vi "GUI_LiquidCrystal.vi"() -> ()   [LabVIEW 2020]
uses:
  Shared/GUI_Template/GUI_master/tcp_new_data_event.ctl
  Shared/GUI_Template/GUI_master/tcp new data cluster.ctl
panel:
  out "Film in place?":bool
  in  "User Threshold":dbl
  in  "MaxCounts::1":dbl caption="Max Counts" min=0.0 max=999999999.0
  in  "Stop":bool
  out "tcp data event":T1
  out "error IO 2":errorcluster
  in  "GUIdevice 1":string="P2-HeatCamPost"
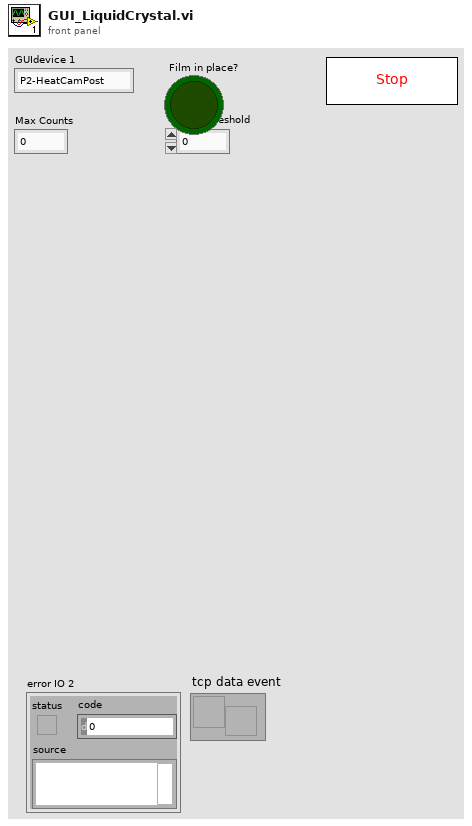
[diagram p1: front panel]
types:
  T1 = typedef "tcp_new_data_event.ctl" = refnum<user-event>
  T2 = typedef "tcp new data cluster.ctl" = cluster{"EventEnum":enum16{"new data", "connection status update"}, "Device name":string}
  T3 = enum32{"Invalid", "Standard", "Closed", "Hidden", "Minimized", "Maximized"}
  T4 = enum32{"invalid app kind", "Development System", "Run Time System", "Student Edition", "Embedded LabVIEW", "Evaluation", "Custom"}
  T5 = cluster{"Core":cluster{"Current VI Reference":refnum<vi>, "Close Panel on Exit?":bool}}
  T6 = cluster{"Current VI Reference":refnum<vi>, "Close Panel on Exit?":bool}
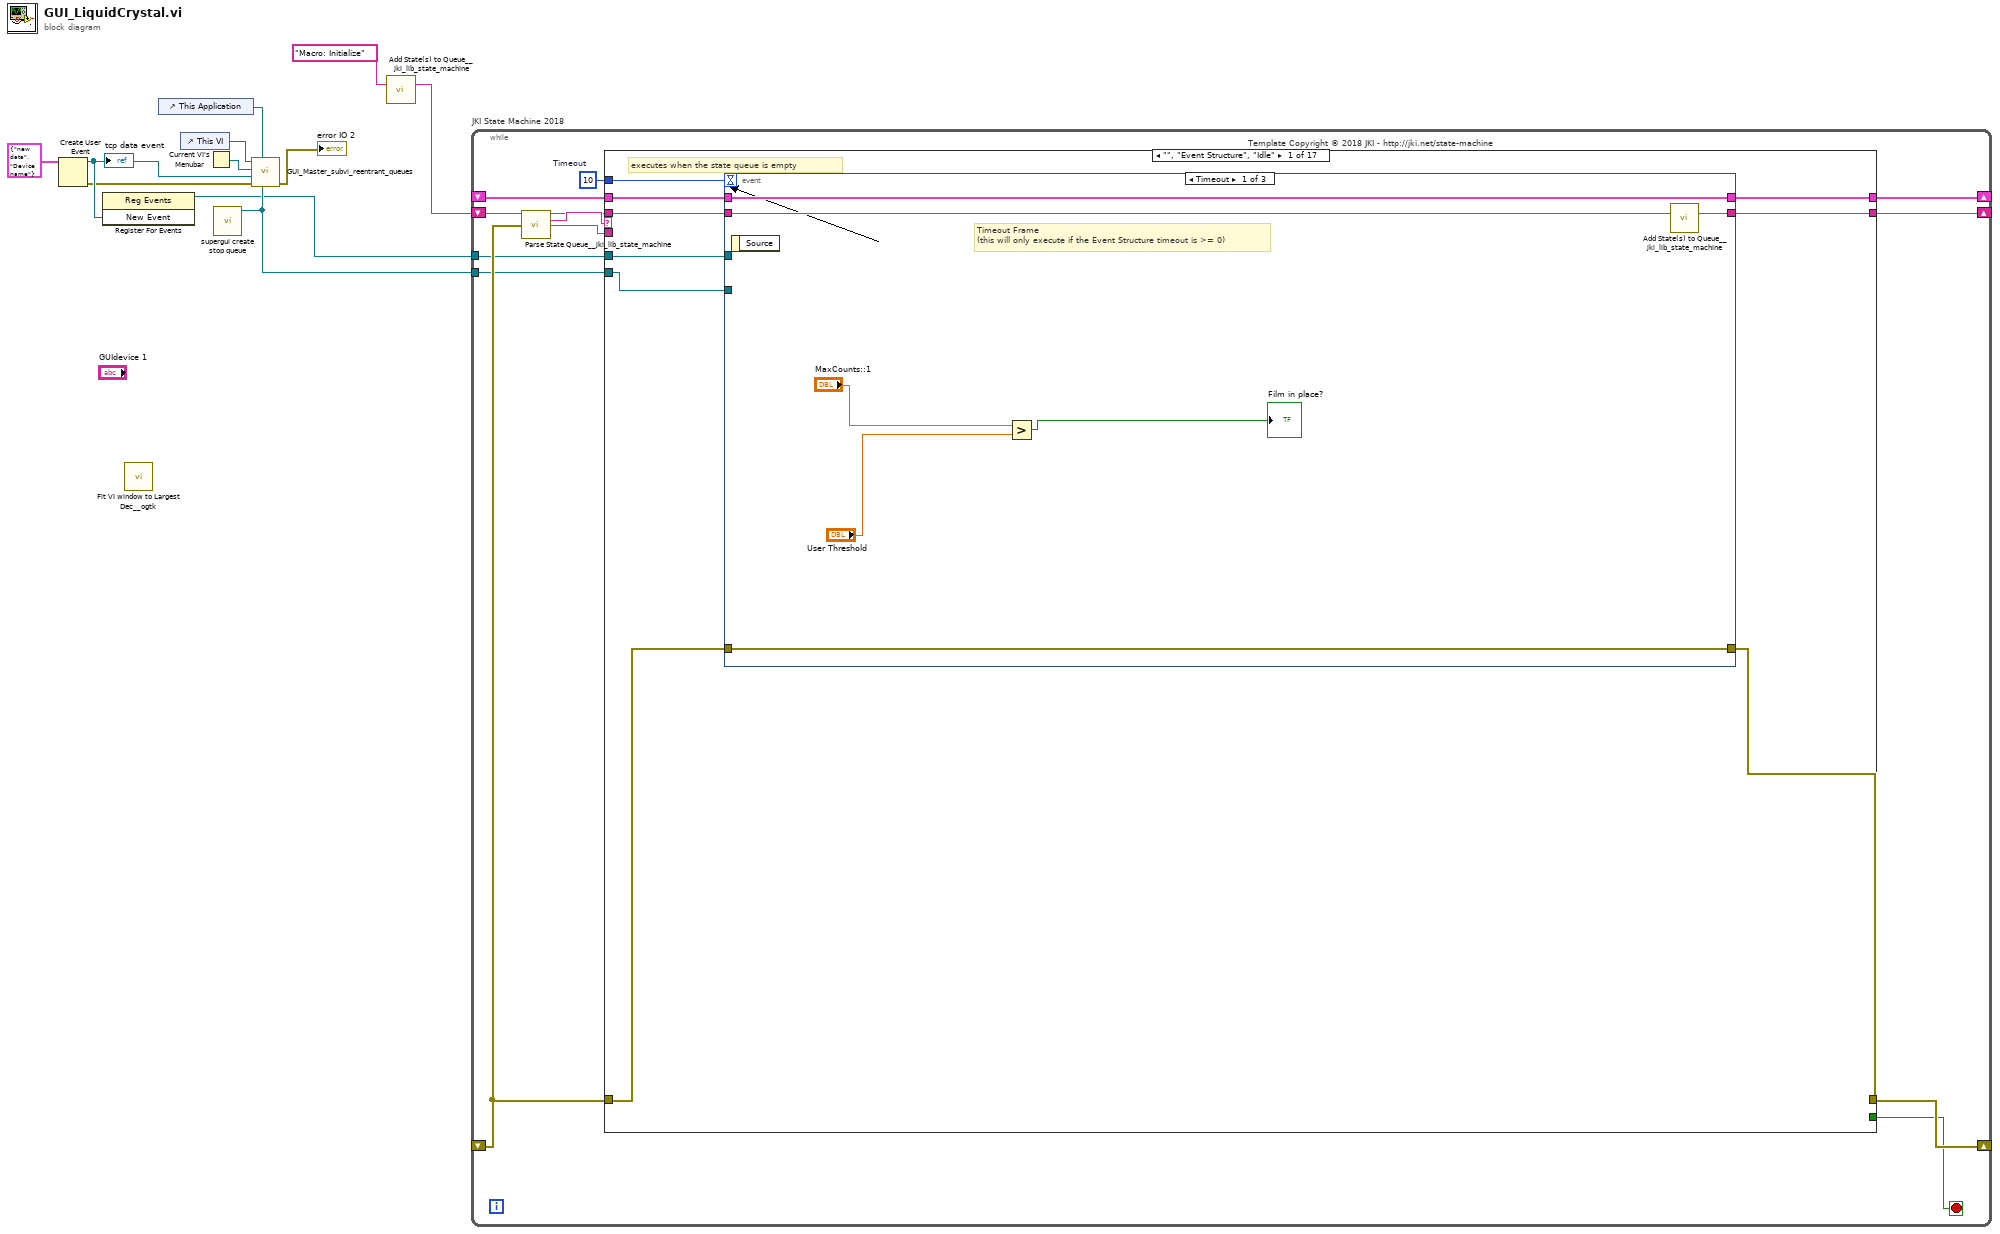
[diagram p0: block diagram]
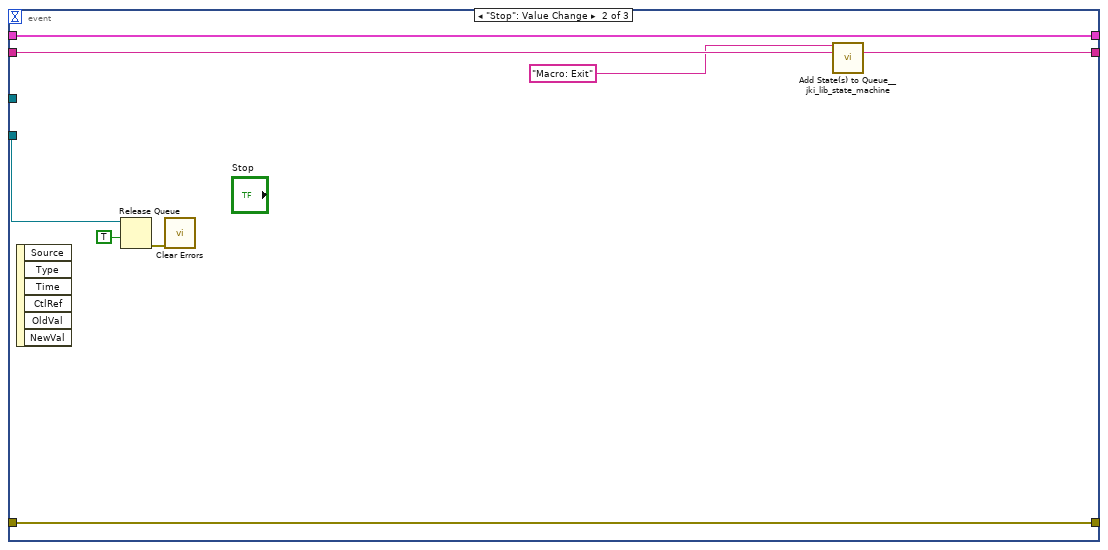
[diagram p2: hidden frame]
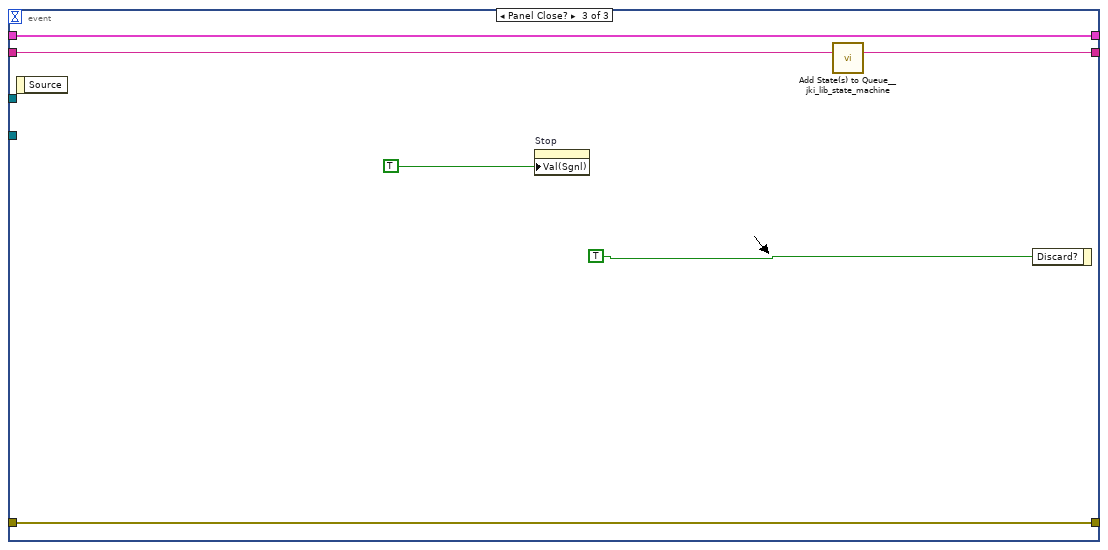
[diagram p3: hidden frame]
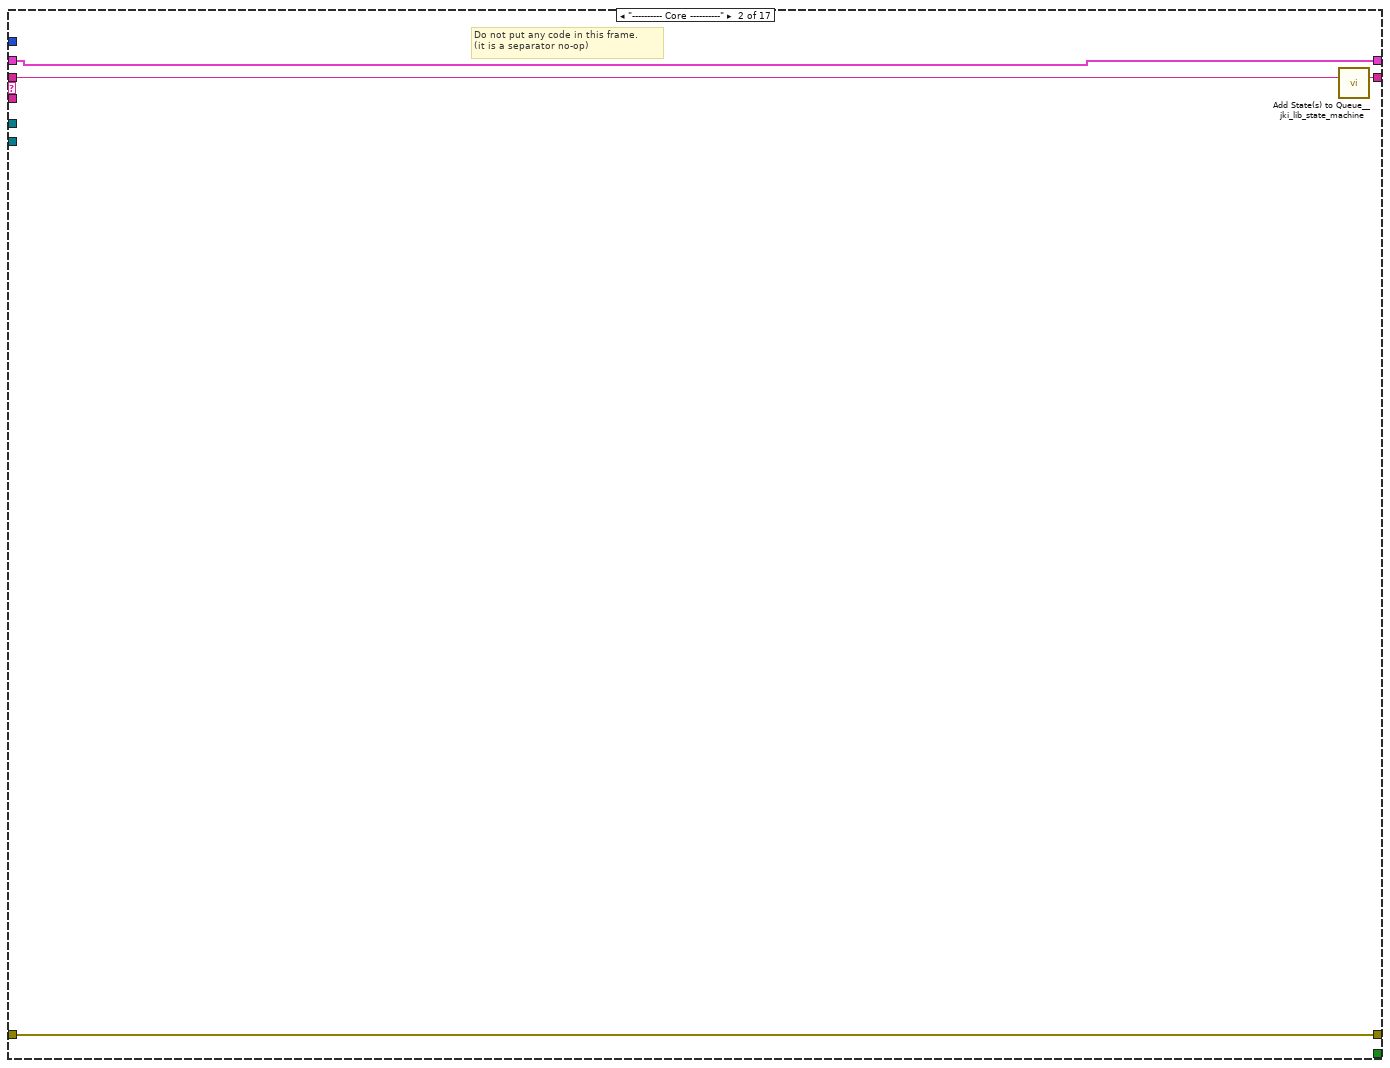
[diagram p4: hidden frame]
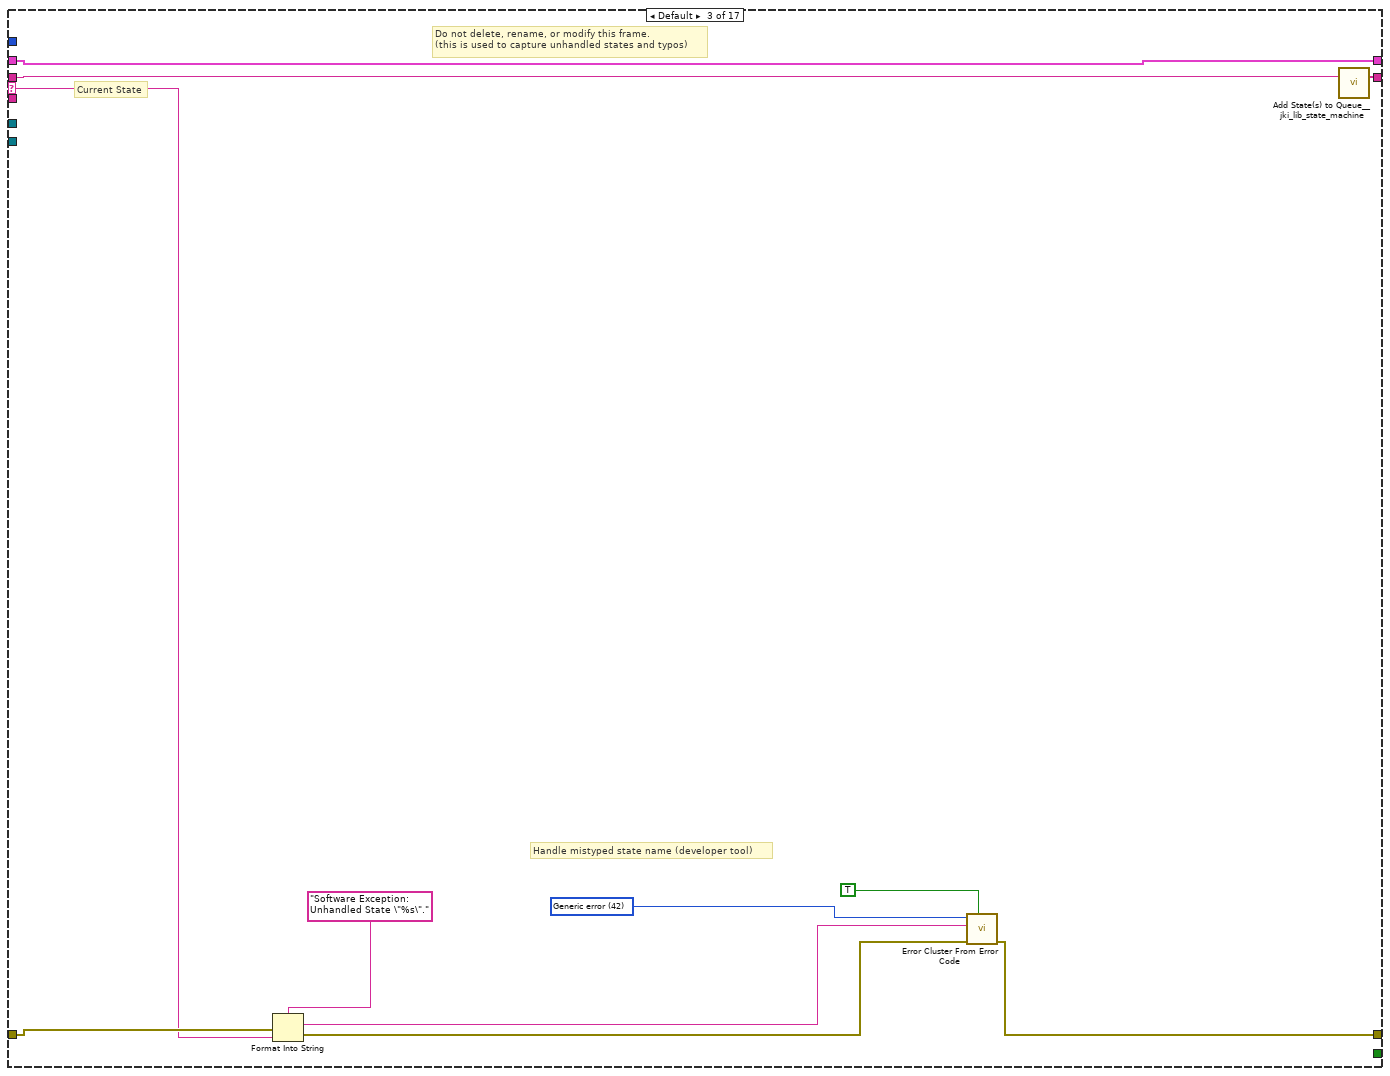
[diagram p5: hidden frame]
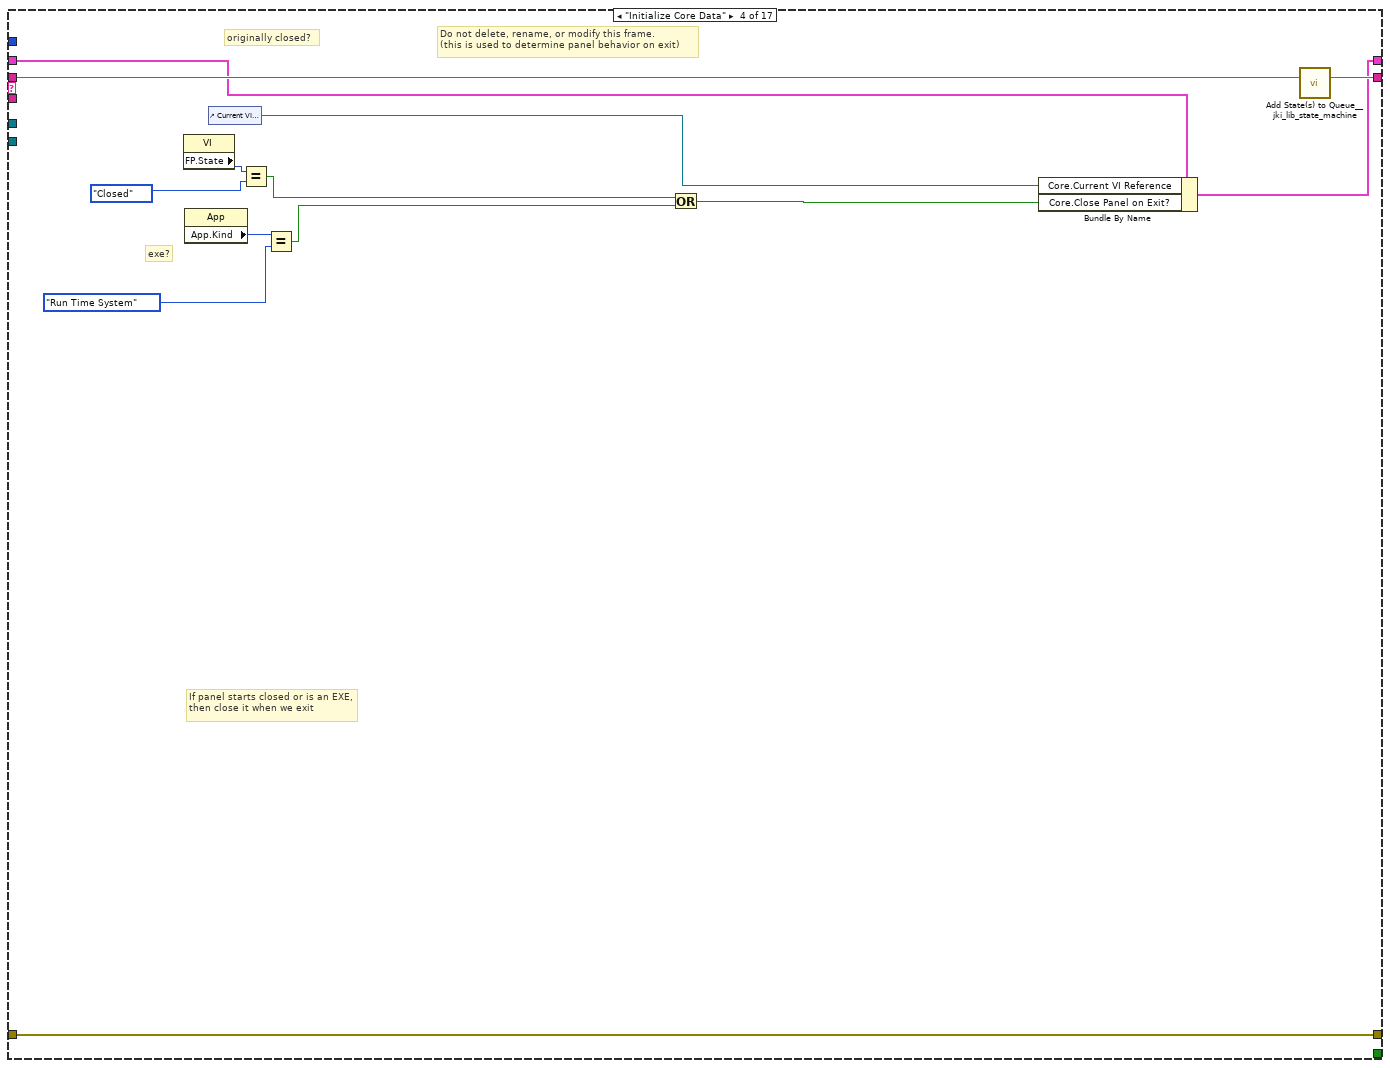
[diagram p6: hidden frame]
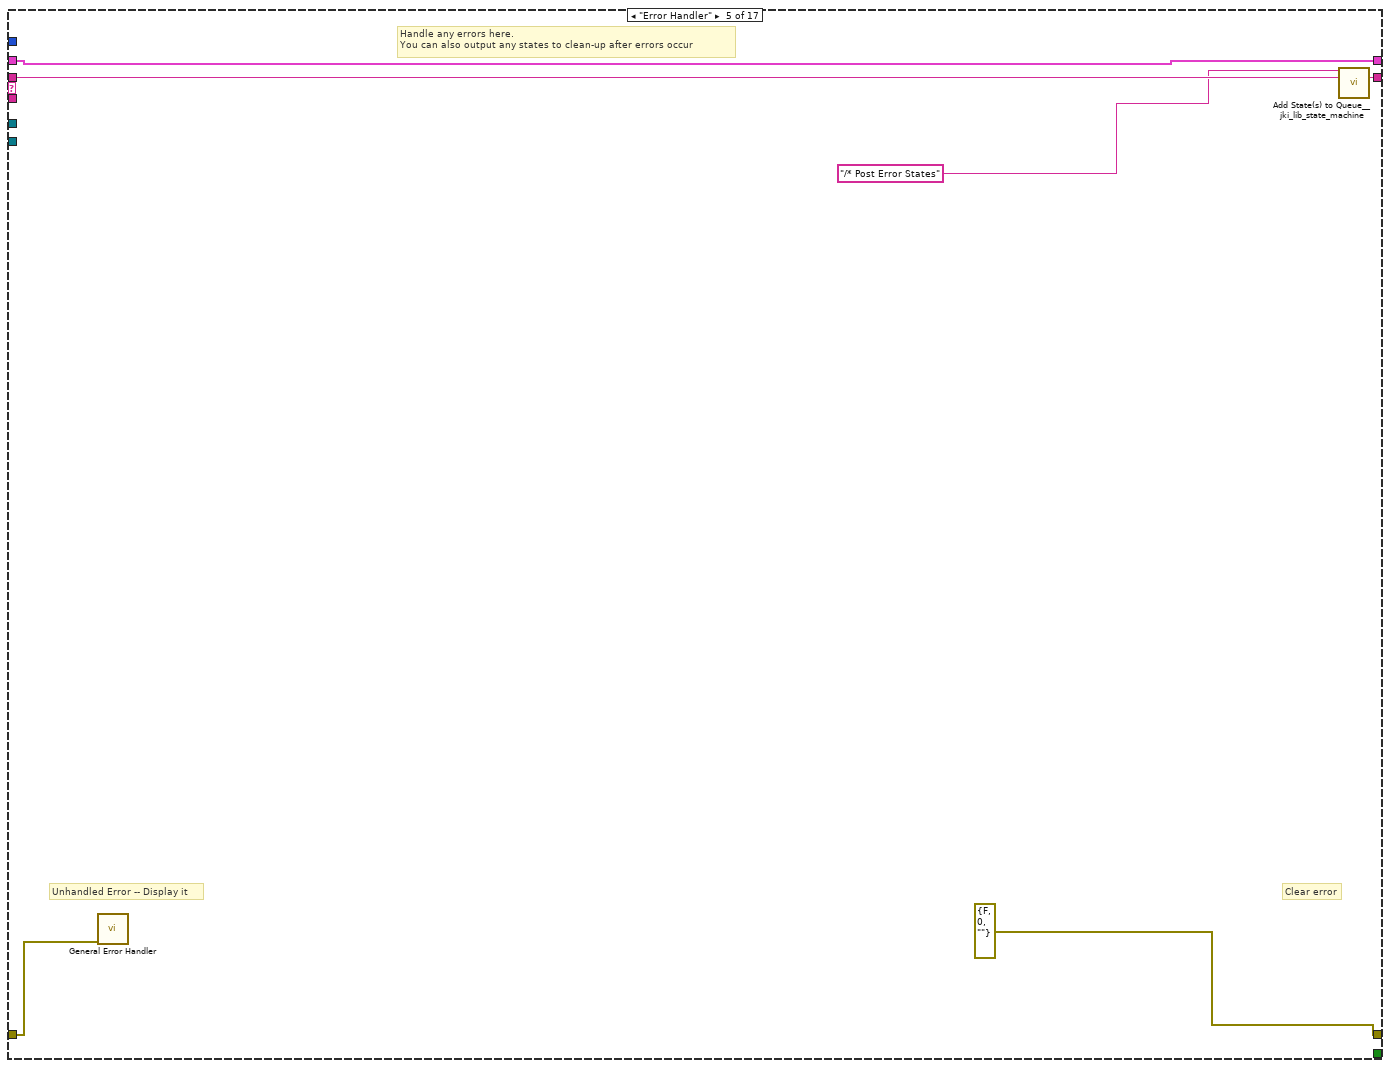
[diagram p7: hidden frame]
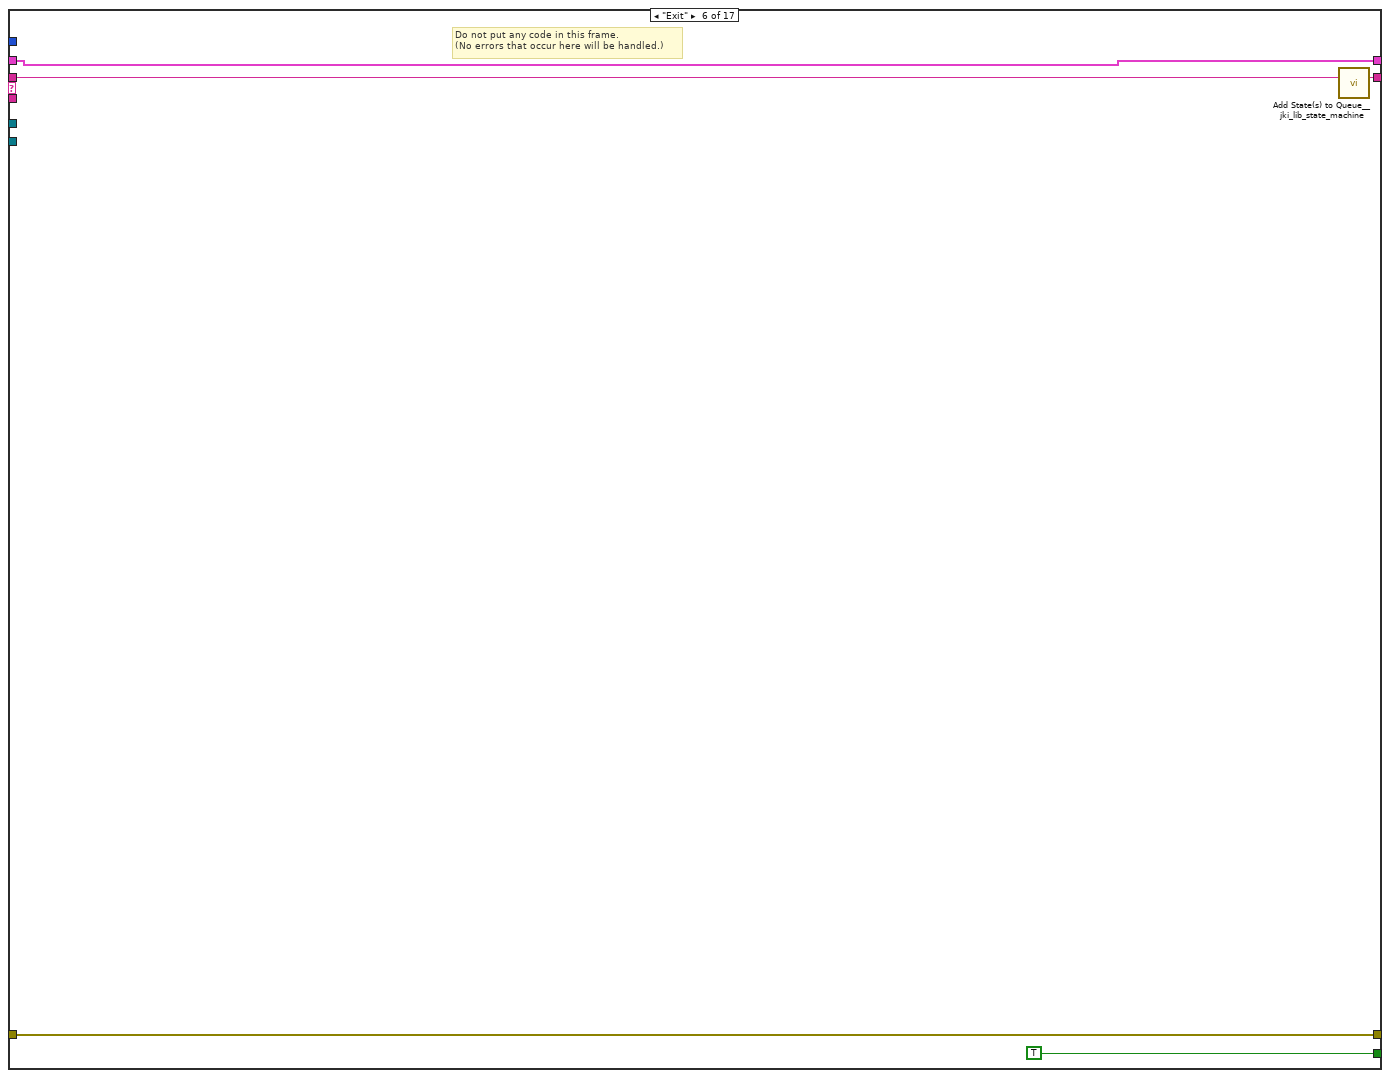
[diagram p8: hidden frame]
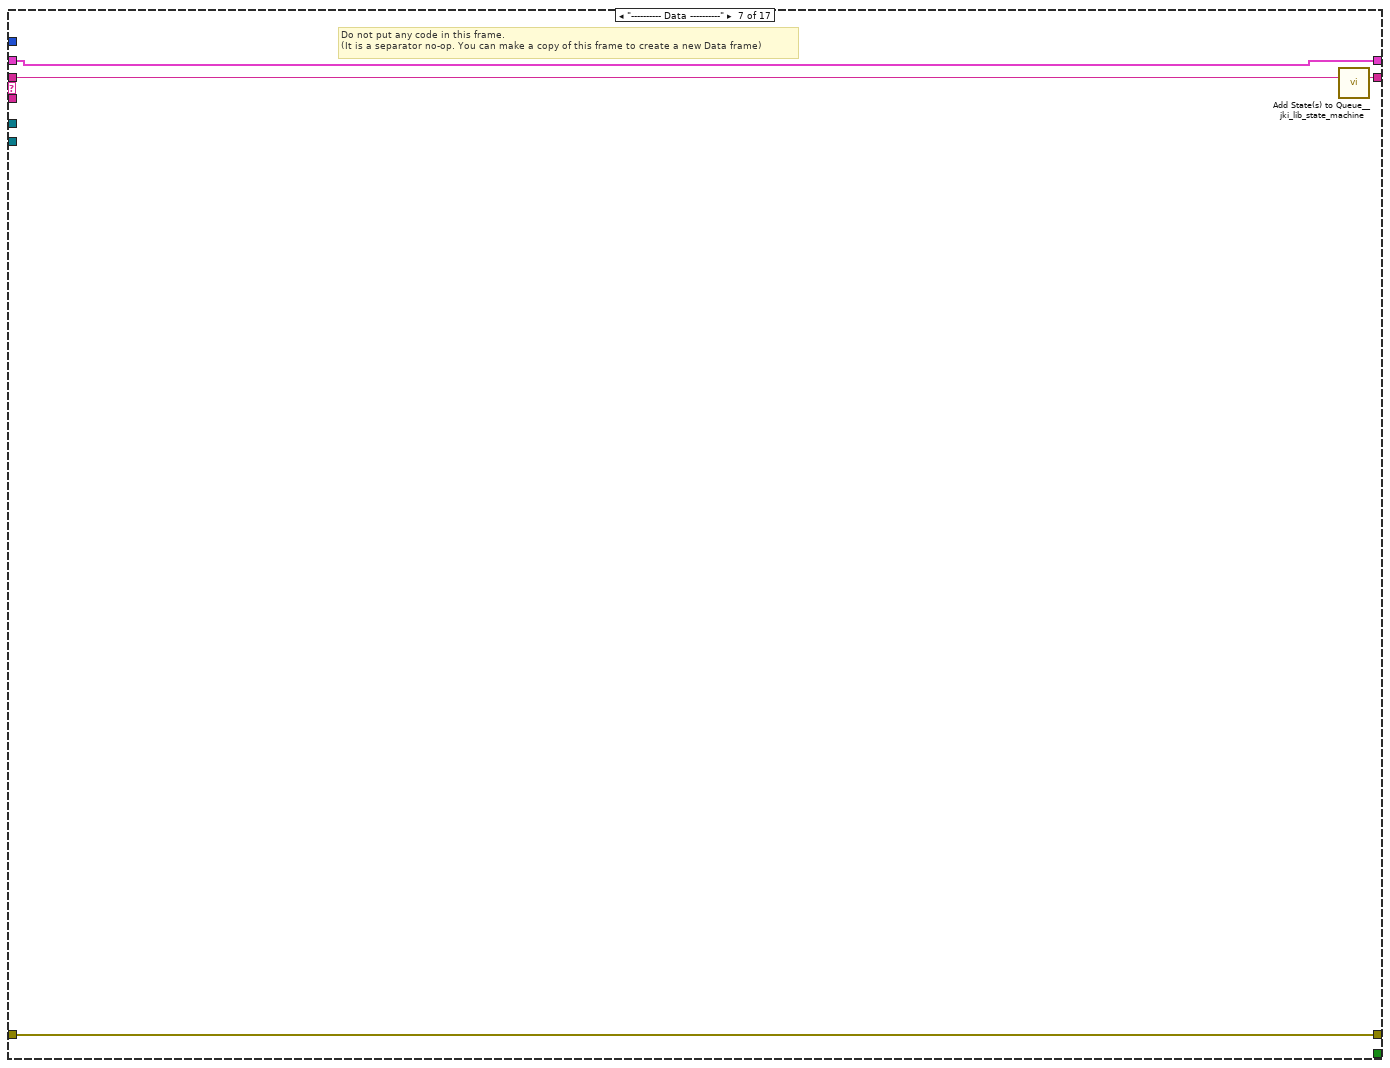
[diagram p9: hidden frame]
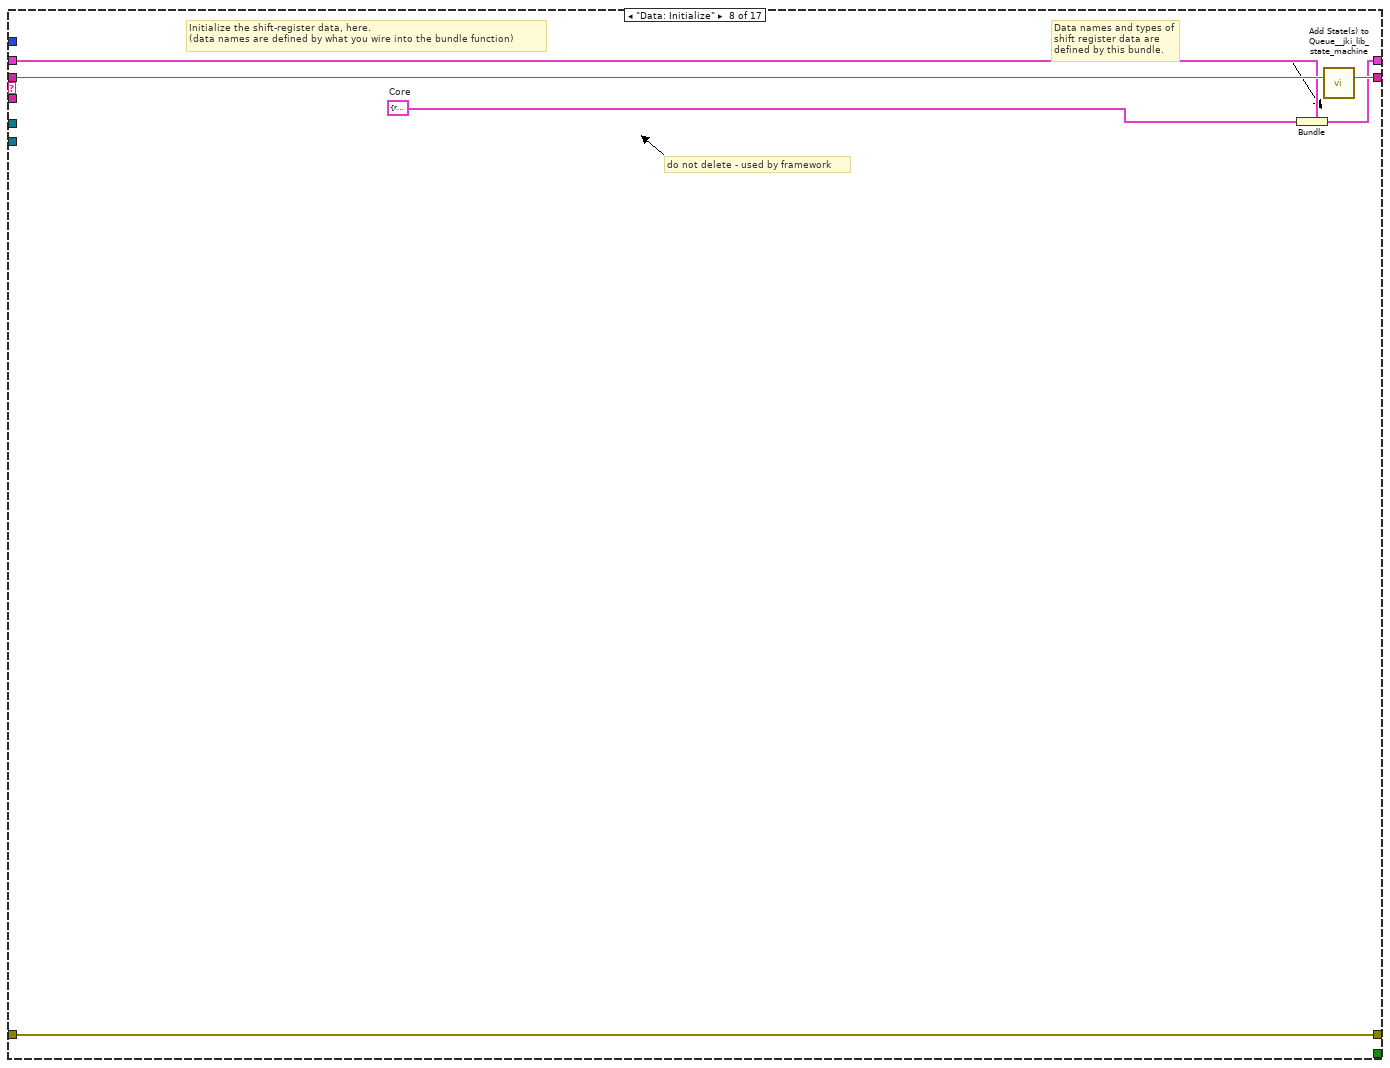
[diagram p10: hidden frame]
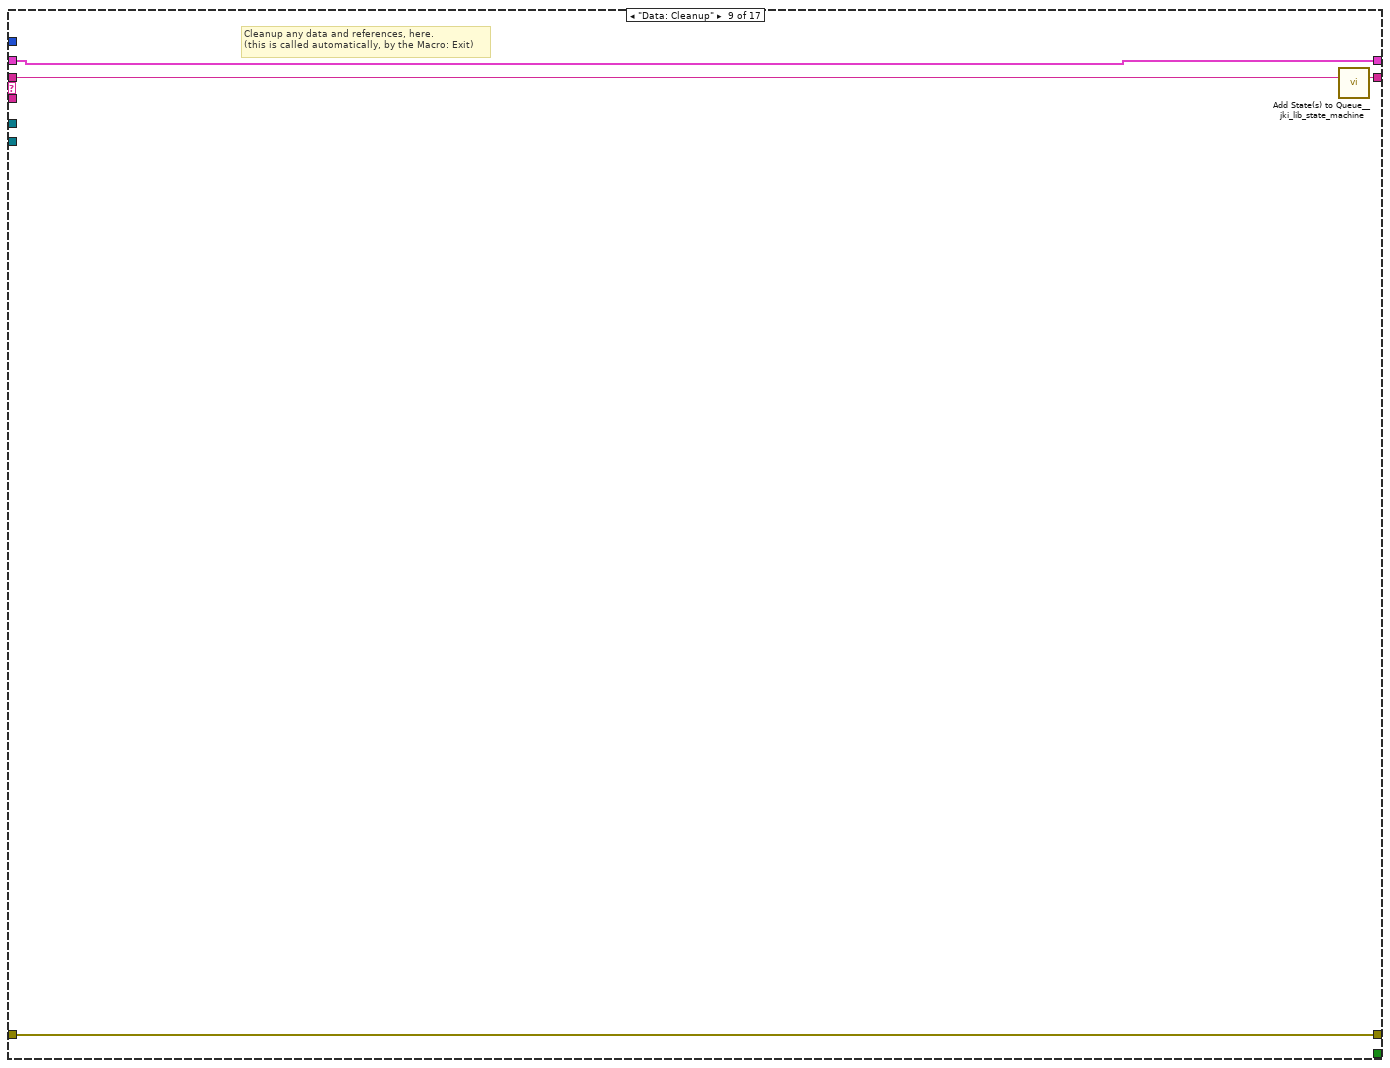
[diagram p11: hidden frame]
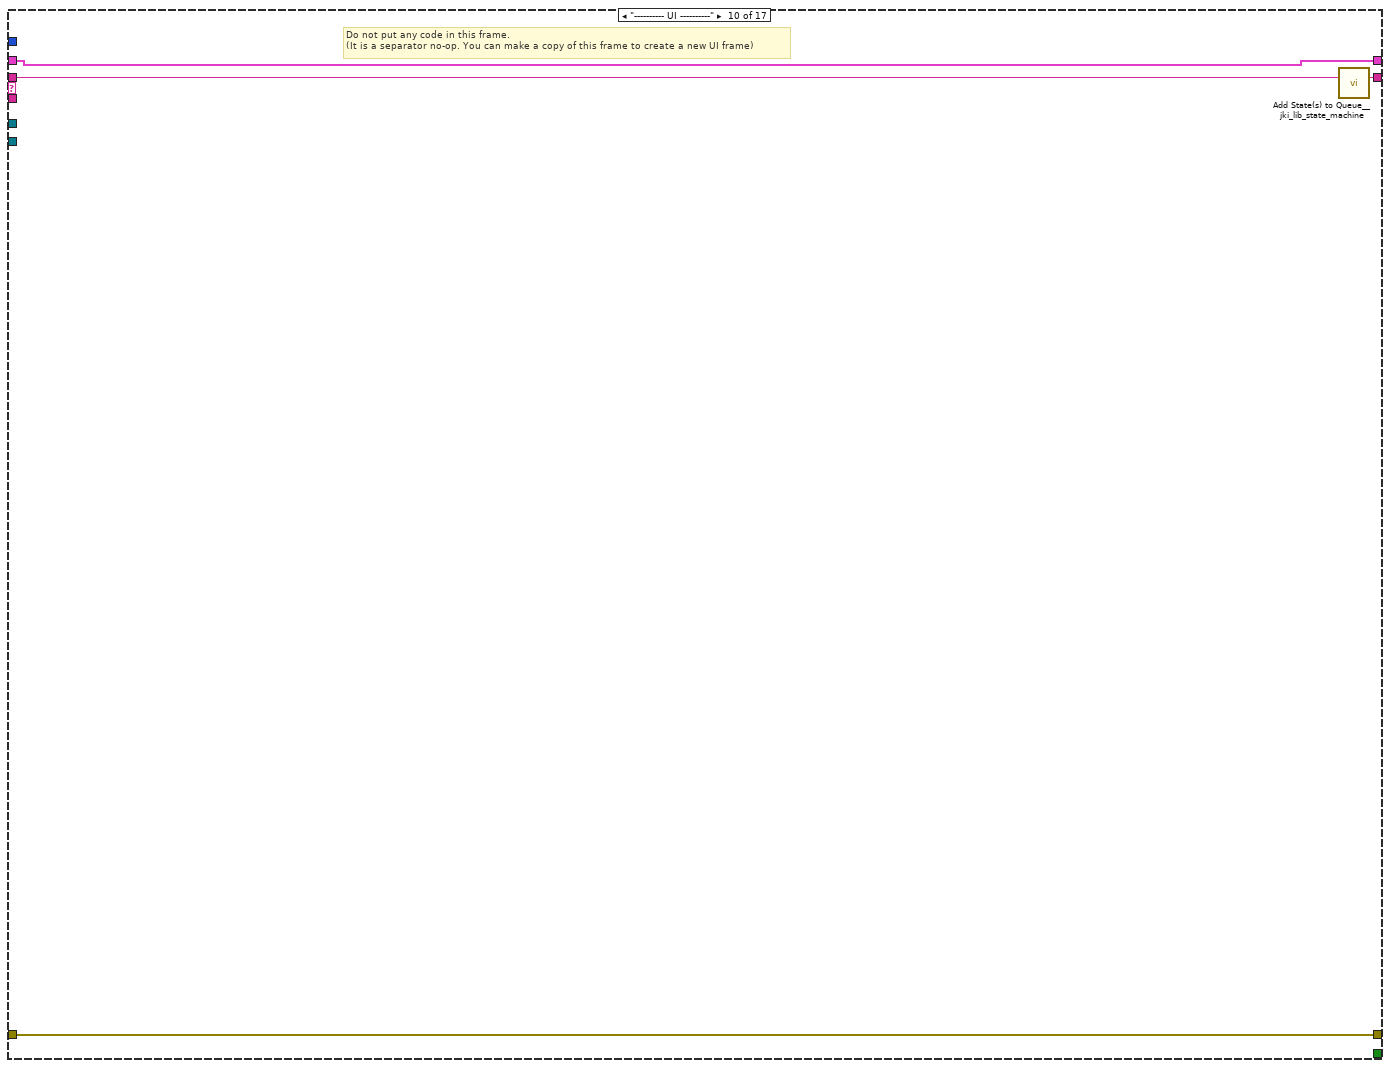
[diagram p12: hidden frame]
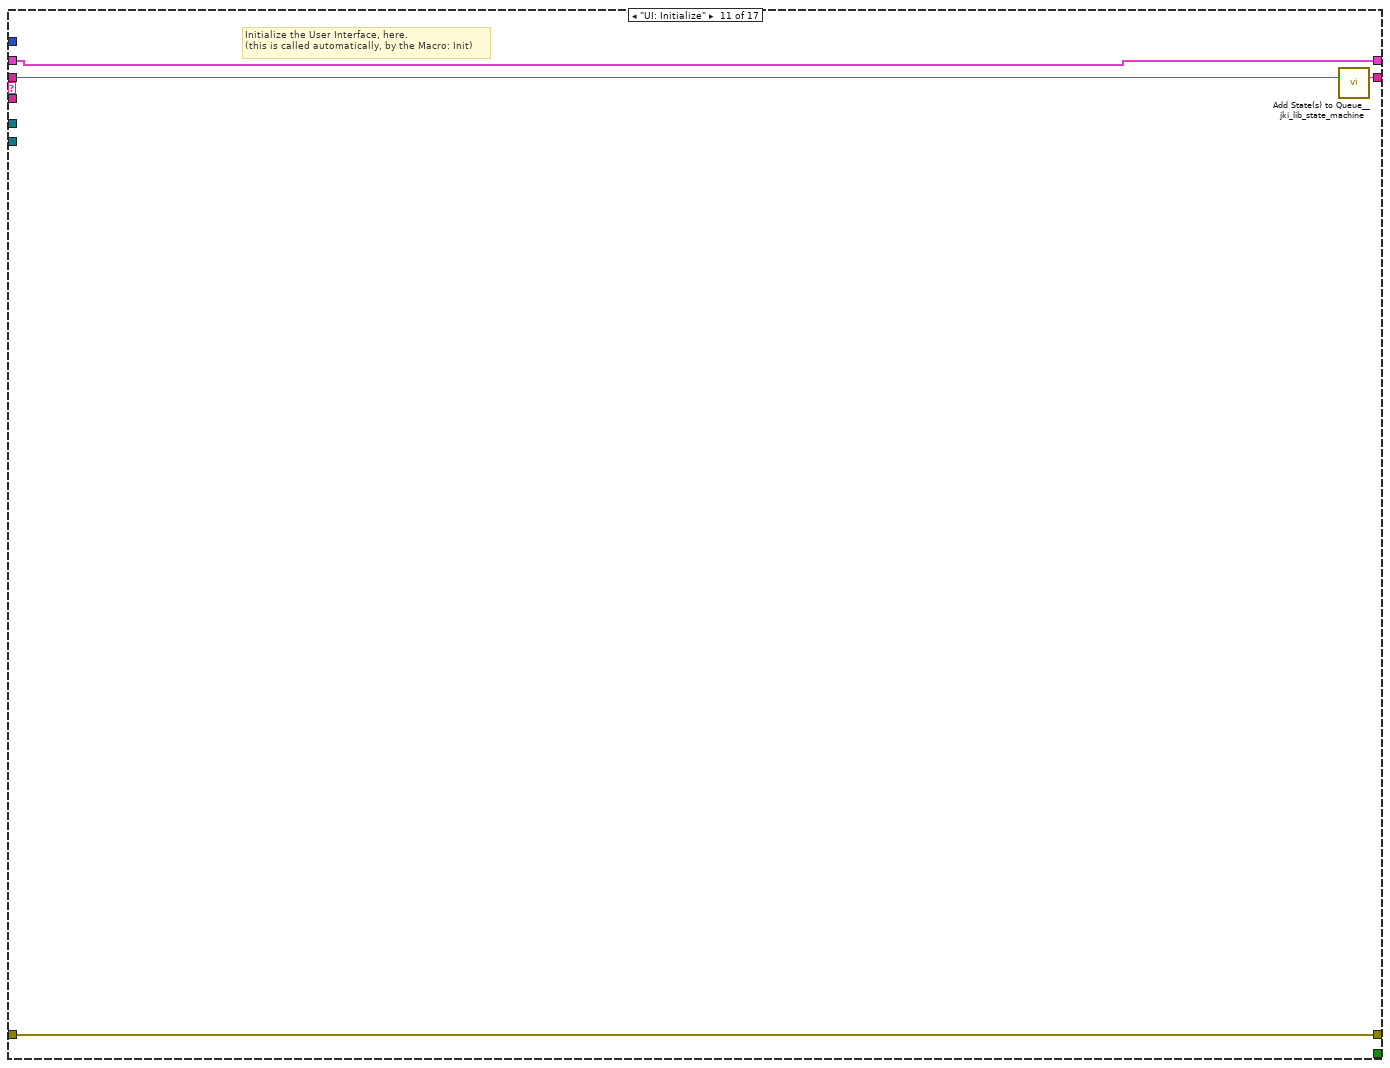
[diagram p13: hidden frame]
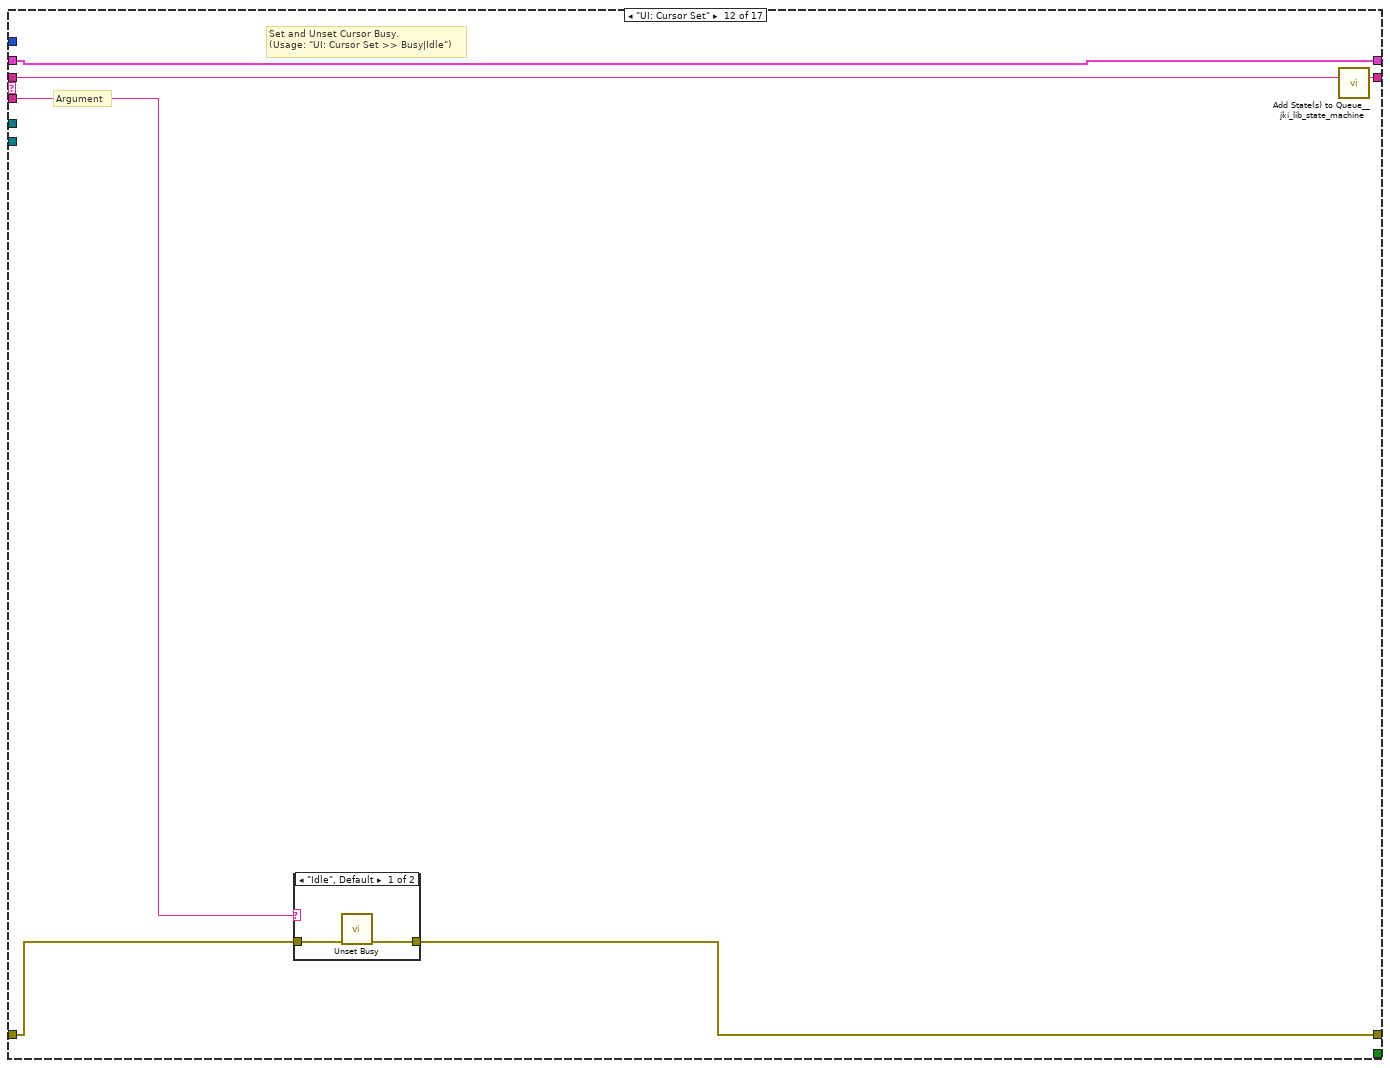
[diagram p14: hidden frame]
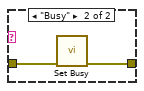
[diagram p15: hidden frame]
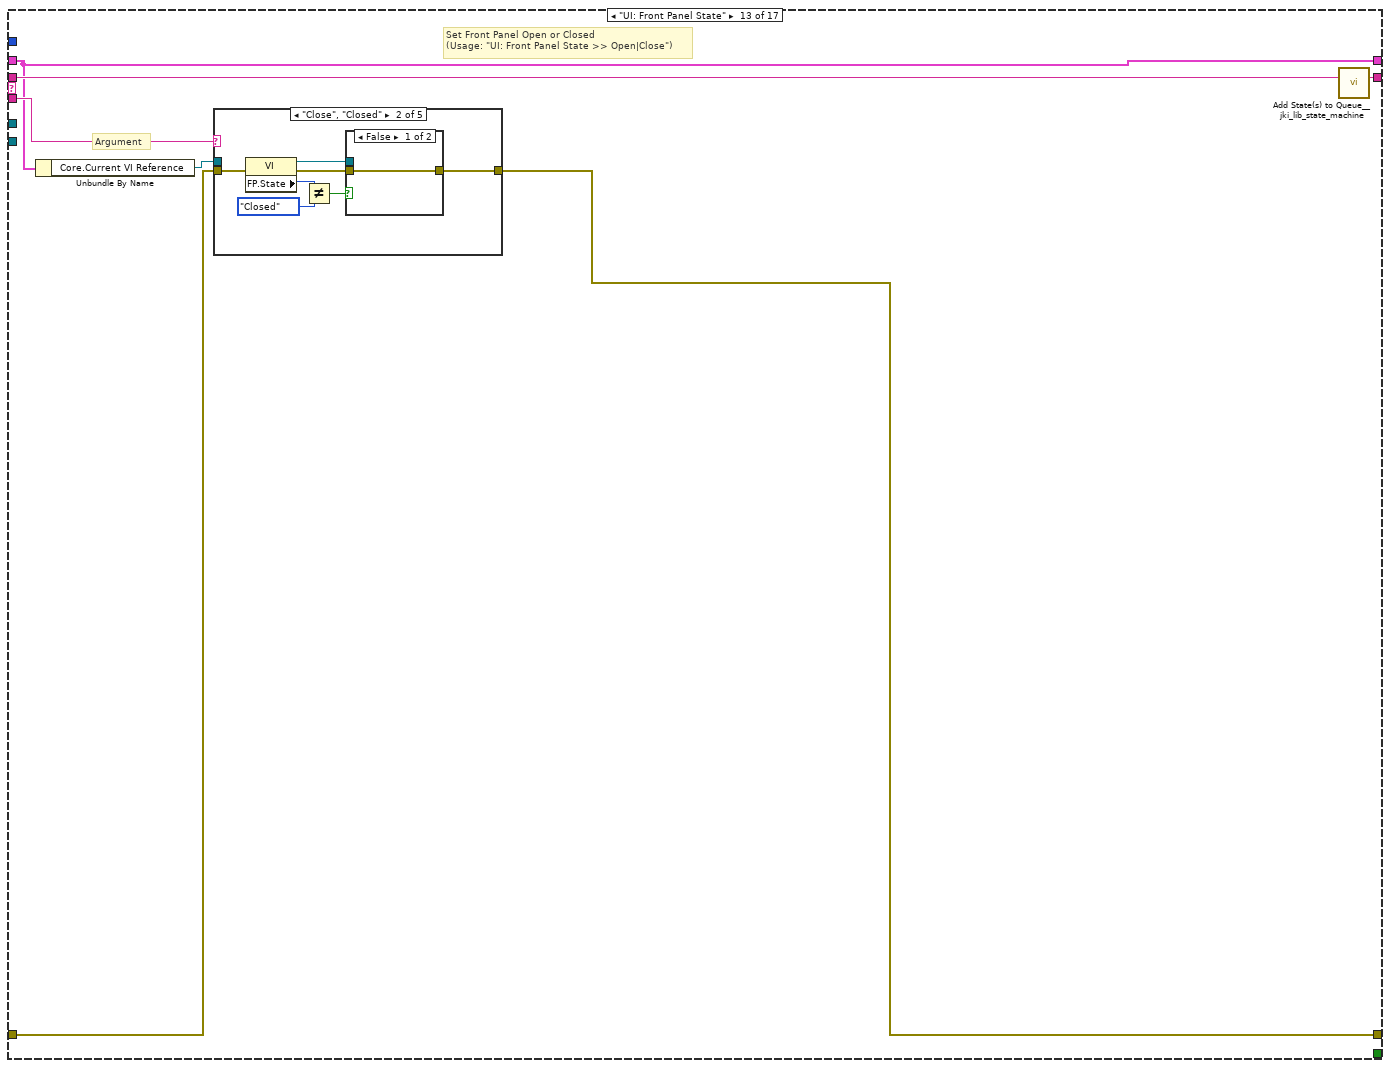
[diagram p16: hidden frame]
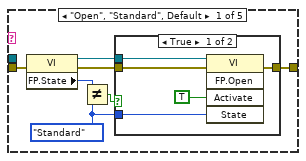
[diagram p17: hidden frame]
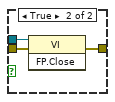
[diagram p19: hidden frame]
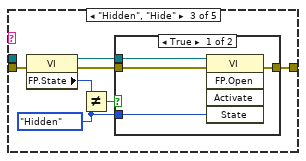
[diagram p20: hidden frame]
diagram:
  n1 = Create User Event(user event datatype=T2 {"EventEnum"=enum."new data", "Device name"="Device name"} ("New Event")) -> (user event=w8:refnum<user-event>, error out=w7:errorcluster)  [unwired: 1 in]
  "tcp data event" <- w8
  n2 = register-events(w8) -> (reference out=w1:refnum<event-registration>)  [unwired: 2 in, 1 out]
  n3 = call <userlib>:"Fit VI window to Largest Dec__ogtk.vi"() -> ()  [unwired: 6 in, 2 out]
  n4 = control-ref of="This Application"() -> (w9:refnum<vi>)
  n5 = control-ref of="This VI"() -> (w4:refnum<vi>)
  n6 = Current VI's Menubar() -> (w5:refnum<k9>)
  n7 = call "supergui create stop queue.vi"() -> ("STOP Queue out"=w2:refnum<queue>)  [unwired: 11 in]
  n8 = call "GUI_Master_subvi_reentrant_queues.vi"("STOP Queue in"=w2, "This Application"=w9, "error in (no error)"=w7, "tcp data event"=w8, "Caller menu reference"=w5, "Caller VI ref"=w4) -> ("error out"=→"error IO 2":errorcluster)  [unwired: 5 in]
  n9 = call <vilib>:"Add State(s) to Queue__jki_lib_state_machine.vi"("State(s) in (\"\")"="Macro: Initialize") -> ("States Out"=w11:string)  [unwired: 14 in]
  n10 = while "JKI State Machine 2018" {
    shift-right: [w19] -> _
    shift-left: _ -> [w18]
    shift-right: [w21] -> _
    shift-left: _ -> [w16]
    shift-right: [w20] -> _
    shift-left: w11 -> [w22]
    tunnel: w1 -> [w15]
    tunnel: w2 -> [w14]
    stop <- w13 stop-if-true
    w17 = 10  # Timeout
    # "Template Copyright © 2018 JKI - http://jki.net/state-machine"
    n11 = call <vilib>:"Parse State Queue__jki_lib_state_machine.vi"("State Queue"=w22, "Error In (no error)"=w16) -> ("Remaining States"=w12:string, "Current State"=w24:string, "Arguments"=w23:string)  [unwired: 11 in]
    n12 = case shown="\"\", \"Event Structure\", \"Idle\"" w24 {
      selector: w24 -> [_ _ w59 _ _ _ _ _ _ _ _ _ _ _ _ _ _]
      tunnel: w12 -> [w33 w58 w63 w82 w88 w93 w97 w103 w107 w111 w115 w121 w132 w196 w201 w211 w218]
      tunnel: w23 -> [_ _ _ _ _ _ _ _ _ _ _ w116 w127 _ _ _ _]
      tunnel: w18 -> [w31 w55 w61 w70 w85 w91 w94 w98 w105 w108 w113 w119 w126 w193 w198 w208 w215]
      tunnel: [w30 w56 w65 w80 errorcluster {"status"=FALSE, "code"=0, "source"=""} ("error out") w90 w95 w101 w104 w109 w112 w117 w129 w194 w199 w209 w216] -> w21
      tunnel: w16 -> [w29 w56 w64 w80 w84 w90 w95 w101 w104 w109 w112 w118 w130 w194 w199 w209 w216]
      tunnel: [w32 w57 w62 w81 w87 w92 w96 w102 w106 w110 w114 w120 w131 w195 w200 w210 w217] -> w20
      tunnel: [_ _ _ _ _ TRUE _ _ _ _ _ _ _ _ _ _ _] -> w13
      tunnel: [w28 w55 w61 w71 w85 w91 w94 w99 w105 w108 w113 w119 w126 w193 w198 w208 w215] -> w19
      tunnel: w17 -> [w27 _ _ _ _ _ _ _ _ _ _ _ _ _ _ _ _]
      tunnel: w15 -> [w26 _ _ _ _ _ _ _ _ _ _ _ _ _ _ _ _]
      tunnel: w14 -> [w25 _ _ _ _ _ _ _ _ _ _ _ _ _ _ _ _]
      frame "", "Event Structure", "Idle" {
        # "executes when the state queue is empty"
        n13 = event shown="[0] Timeout" {
          selector: _ -> [_ _ _]
          dyn-events: _ -> [_ _ _]
          timeout: w27 -> [_ _ _]
          tunnel: w33 -> [w40 w48 w54]
          tunnel: [w39 w47 w53] -> w32
          tunnel: w31 -> [w38 w45 w51]
          tunnel: [w37 w46 w52] -> w30
          tunnel: w29 -> [w37 w46 w52]
          tunnel: [w38 w45 w51] -> w28
          tunnel: w26 -> [_ _ _]
          tunnel: w25 -> [_ w41 _]
          event Timeout {
            # "Timeout Frame\n(this will only execute if the Event Structure timeout is >= 0)"
            n14 = event-data() -> ()  [unwired: 1 in, 1 out]
            n15 = Greater?(x="MaxCounts::1", y="User Threshold") -> (0:→"Film in place?":bool)
            n16 = call <vilib>:"Add State(s) to Queue__jki_lib_state_machine.vi"("State(s) in (\"\")"=w40) -> ("States Out"=w39:string)  [unwired: 14 in]
          }
          event "Stop": Value Change {
            n17 = event-data() -> ()  [unwired: 1 in, 6 out]
            n18 = Release Queue(queue=w41, force destroy? (F)=TRUE) -> (error out=w43:errorcluster)  [unwired: 1 in, 2 out]
            n19 = call <vilib>:"Clear Errors.vi"("error in (no error)"=w43) -> ()  [unwired: 5 in, 2 out]
            n20 = call <vilib>:"Add State(s) to Queue__jki_lib_state_machine.vi"("State(s) in Front (\"\")"="Macro: Exit", "State(s) in (\"\")"=w48) -> ("States Out"=w47:string)  [unwired: 13 in]
          }
          event Panel Close? {
            n21 = event-data() -> ()  [unwired: 1 in, 1 out]
            n22 = property on="Stop" class="Bool (strict)"("Val(Sgnl)"=TRUE ("stop")) -> ()  [unwired: 2 in, 2 out]
            n23 = call <vilib>:"Add State(s) to Queue__jki_lib_state_machine.vi"("State(s) in (\"\")"=w54) -> ("States Out"=w53:string)  [unwired: 14 in]
            n24 = event-data("Discard?"=TRUE) -> ()  [unwired: 1 in, 1 out]
          }
        }
      }
      frame "---------- Core ----------" {
        # "Do not put any code in this frame.\n(it is a separator no-op)"
        n25 = call <vilib>:"Add State(s) to Queue__jki_lib_state_machine.vi"("State(s) in (\"\")"=w58) -> ("States Out"=w57:string)  [unwired: 14 in]
      }
      frame Default {
        w68 = 42 items=["No error", "Argument error", "Memory is full", "Out of zone", "End of file", "File already open", "Generic file I/O error", "File not found", "File permission error", "Disk is full", "Duplicate path", "Too many files open", "System feature not enabled", "Resource file not found", "Cannot add resource", "Resource not found", "Image not found", "Image memory error", "Pen does not exist", "Config type invalid", "Config token not found", "Config parse error", "Config memory error", "Bad external code format", "Bad external code offset", "External code not present", "Null window", "Destroy window error", "Null menu", "Print aborted", "Bad print record", "Print driver error", "Windows error during printing", "Memory error during printing", "Print dialog error", "Generic print error", "Invalid device refnum", "Device not found", "Device parameter error", "Device unit error", "Cannot open device", "Device call aborted", "Generic error", "Cancelled by user", "Object ID too low", "Object ID too high", "Object not in heap", "Unknown heap", "Unknown object (invalid DefProc)", "Unknown object (DefProc not in table)", "Message out of range", "Invalid (null) method", "Unknown message", "Manager call not supported", "Bad address", "Network operation in progress", "Network operation timed out", "Connection is busy", "Network attribute not supported", "Network error", "Address in use", "System out of memory", "Connection aborted", "Connection refused", "Not connected", "Already connected", "Connection closed", "Initialization error (interapplication manager)", "Bad occurrence", "Wait on unbound occurrence handler", "Occurrence queue overflow", "Datalog type conflict", "Unused", "Unrecognized type (interapplication manager)", "Memory corrupt", "Failed to make temporary DLL", "Old CIN version", "Drag socket not found", "Failed to load drop-object", "Failed to register OLE object", "Failed to release OLE object", "Format specifier type mismatch", "Unknown format specifier", "Too few format specifiers", "Too many format specifiers", "Scan failed", "Newer CIN version", "Error converting to variant", "Runtime menu error", "Password tampered", "Variant attribute not found", "Incompatible variant data type", "Event data is not available", "Event Store is not present", "Occurrence is not found", "Event Queue is not created", "Event info is not available", "Refnum passed is NULL", "Error retrieving Class GUID", "Error retrieving CoClass GUID", "Error retrieving TypeLib GUID.", "Bad built application magic bytes.", "Specific driver is different from the specific driver associated with the Logical Name.", "There is no session opened to the class driver.", "Max Error", "MAX - Error with config objects", "MAX - Error loading configuration", "MAX - Group not supported"]
        # "Current State"
        # "Do not delete, rename, or modify this frame.\n(this is used to capture unhandled states and typos)"
        # "Handle mistyped state name (developer tool)"
        n26 = Format Into String(format string="Software Exception: Unhandled State \"%s\"." ("message"), error in=w64, w59) -> (resulting string=w67:string, error out=w66:errorcluster)  [unwired: 1 in]
        n27 = call <vilib>:"Error Cluster From Error Code.vi"("show call chain? (False)"=TRUE, "error in (no error)"=w66, "error message (\"\")"=w67, "error code (0)"=w68) -> ("error out"=w65:errorcluster)  [unwired: 5 in]
        n28 = call <vilib>:"Add State(s) to Queue__jki_lib_state_machine.vi"("State(s) in (\"\")"=w63) -> ("States Out"=w62:string)  [unwired: 14 in]
      }
      frame "Initialize Core Data" {
        # "Do not delete, rename, or modify this frame.\n(this is used to determine panel behavior on exit)"
        # "originally closed?"
        # "exe?"
        # "If panel starts closed or is an EXE, then close it when we exit"
        n29 = property class="VI"() -> ("FP.State"=w74:T3)  [unwired: 2 in, 2 out]
        n30 = property class="App"() -> ("App.Kind"=w79:T4)  [unwired: 2 in, 2 out]
        n31 = control-ref of="Current VI Reference"() -> (w75:refnum<vi>)
        n32 = Equal?(x=w74, y=T3."Closed" ("Front Panel Window:State")) -> (x = y?=w72:bool)
        n33 = Equal?(x=w79, y=T4."Run Time System" ("Application:Kind")) -> (x = y?=w77:bool)
        n34 = Or(x=w72, y=w77) -> (x .or. y?=w76:bool)
        n35 = Bundle By Name(cluster=w70, "Core.Current VI Reference"=w75, "Core.Close Panel on Exit?"=w76) -> (w71:T5)
        n36 = call <vilib>:"Add State(s) to Queue__jki_lib_state_machine.vi"("State(s) in (\"\")"=w82) -> ("States Out"=w81:string)  [unwired: 14 in]
      }
      frame "Error Handler" {
        # "Unhandled Error -- Display it"
        # "Handle any errors here.\nYou can also output any states to clean-up after errors occur"
        # "Clear error"
        n37 = call <vilib>:"General Error Handler.vi"("error in (no error)"=w84) -> ()  [unwired: 10 in, 5 out]
        n38 = call <vilib>:"Add State(s) to Queue__jki_lib_state_machine.vi"("State(s) in Front (\"\")"="/* Post Error States", "State(s) in (\"\")"=w88) -> ("States Out"=w87:string)  [unwired: 13 in]
      }
      frame "Exit" {
        # "Do not put any code in this frame.\n(No errors that occur here will be handled.)"
        n39 = call <vilib>:"Add State(s) to Queue__jki_lib_state_machine.vi"("State(s) in (\"\")"=w93) -> ("States Out"=w92:string)  [unwired: 14 in]
      }
      frame "---------- Data ----------" {
        # "Do not put any code in this frame.\n(It is a separator no-op. You can make a copy of this frame to create a new Data frame)"
        n40 = call <vilib>:"Add State(s) to Queue__jki_lib_state_machine.vi"("State(s) in (\"\")"=w97) -> ("States Out"=w96:string)  [unwired: 14 in]
      }
      frame "Data: Initialize" {
        w100 = T6 {"Current VI Reference"=refnum, "Close Panel on Exit?"=FALSE}  # Core
        # "do not delete - used by framework"
        # "Data names and types of shift register data are defined by this bundle."
        # "Initialize the shift-register data, here.\n(data names are defined by what you wire into the bundle function)"
        n41 = Bundle(cluster=w98, "Core"=w100) -> (w99:T5)
        n42 = call <vilib>:"Add State(s) to Queue__jki_lib_state_machine.vi"("State(s) in (\"\")"=w103) -> ("States Out"=w102:string)  [unwired: 14 in]
      }
      frame "Data: Cleanup" {
        # "Cleanup any data and references, here.\n(this is called automatically, by the Macro: Exit)"
        n43 = call <vilib>:"Add State(s) to Queue__jki_lib_state_machine.vi"("State(s) in (\"\")"=w107) -> ("States Out"=w106:string)  [unwired: 14 in]
      }
      frame "---------- UI ----------" {
        # "Do not put any code in this frame.\n(It is a separator no-op. You can make a copy of this frame to create a new UI frame)"
        n44 = call <vilib>:"Add State(s) to Queue__jki_lib_state_machine.vi"("State(s) in (\"\")"=w111) -> ("States Out"=w110:string)  [unwired: 14 in]
      }
      frame "UI: Initialize" {
        # "Initialize the User Interface, here.\n(this is called automatically, by the Macro: Init)"
        n45 = call <vilib>:"Add State(s) to Queue__jki_lib_state_machine.vi"("State(s) in (\"\")"=w115) -> ("States Out"=w114:string)  [unwired: 14 in]
      }
      frame "UI: Cursor Set" {
        # "Argument"
        # "Set and Unset Cursor Busy.\n(Usage: \"UI: Cursor Set >> Busy|Idle\")"
        n46 = case shown="\"Idle\", Default" w116 {
          tunnel: w118 -> [w123 w125]
          tunnel: [w122 w124] -> w117
          frame "Idle", Default {
            n47 = call <vilib>:"Unset Busy.vi"("error in (no error)"=w123) -> ("error out"=w122:errorcluster)  [unwired: 10 in]
          }
          frame "Busy" {
            n48 = call <vilib>:"Set Busy.vi"("error in (no error)"=w125) -> ("error out"=w124:errorcluster)  [unwired: 9 in, 1 out]
          }
        }
        n49 = call <vilib>:"Add State(s) to Queue__jki_lib_state_machine.vi"("State(s) in (\"\")"=w121) -> ("States Out"=w120:string)  [unwired: 14 in]
      }
      frame "UI: Front Panel State" {
        # "Argument"
        # "Set Front Panel Open or Closed\n(Usage: \"UI: Front Panel State >> Open|Close\")"
        n50 = Unbundle By Name(w126) -> ("Core.Current VI Reference"=w128:refnum<vi>)
        n51 = case shown="\"Close\", \"Closed\"" w127 {
          tunnel: w130 -> [w138 w151 w162 w174 w186]
          tunnel: [w139 w152 w163 w175 w187] -> w129
          tunnel: w128 -> [_ _ _ _ _]
          frame "Open", "Standard", Default {
            w133 = T3."Standard" ("State")
            n52 = property class="VI"(error in=w138) -> (reference out=w136:refnum<vi>, error out=w137:errorcluster, "FP.State"=w135:T3)  [unwired: 1 in]
            n53 = Not Equal?(x=w135, y=w133) -> (x != y?=w134:bool)
            n54 = case shown="True" w134 {
              tunnel: [w143 w145] -> w139
              tunnel: w137 -> [w142 w145]
              tunnel: w136 -> [w141 _]
              tunnel: w133 -> [w140 _]
              frame True {
                n55 = invoke class="VI" method="FP.Open"(reference=w141, error in=w142, "Activate"=TRUE, "State"=w140) -> (error out=w143:errorcluster)  [unwired: 1 in, 4 out]
              }
              frame False {
              }
            }
          }
          frame "Close", "Closed" {
            n56 = property class="VI"(error in=w151) -> (reference out=w149:refnum<vi>, error out=w150:errorcluster, "FP.State"=w147:T3)  [unwired: 1 in]
            n57 = Not Equal?(x=w147, y=T3."Closed" ("Front Panel Window:State")) -> (x != y?=w146:bool)
            n58 = case shown="False" w146 {
              tunnel: [w153 w156] -> w152
              tunnel: w150 -> [w153 w155]
              tunnel: w149 -> [_ w154]
              frame False {
              }
              frame True {
                n59 = invoke class="VI" method="FP.Close"(reference=w154, error in=w155) -> (error out=w156:errorcluster)  [unwired: 1 in, 2 out]
              }
            }
          }
          frame "Hidden", "Hide" {
            w157 = T3."Hidden" ("State")
            n60 = property class="VI"(error in=w162) -> (reference out=w160:refnum<vi>, error out=w161:errorcluster, "FP.State"=w159:T3)  [unwired: 1 in]
            n61 = Not Equal?(x=w159, y=w157) -> (x != y?=w158:bool)
            n62 = case shown="True" w158 {
              tunnel: [w167 w168] -> w163
              tunnel: w161 -> [w166 w168]
              tunnel: w160 -> [w165 _]
              tunnel: w157 -> [w164 _]
              frame True {
                n63 = invoke class="VI" method="FP.Open"(reference=w165, error in=w166, "State"=w164) -> (error out=w167:errorcluster)  [unwired: 2 in, 4 out]
              }
              frame False {
              }
            }
          }
          frame "Minimize", "Minimized" {
            w169 = T3."Minimized" ("State")
            n64 = property class="VI"(error in=w174) -> (reference out=w172:refnum<vi>, error out=w173:errorcluster, "FP.State"=w171:T3)  [unwired: 1 in]
            n65 = Not Equal?(x=w171, y=w169) -> (x != y?=w170:bool)
            n66 = case shown="True" w170 {
              tunnel: [w179 w180] -> w175
              tunnel: w173 -> [w178 w180]
              tunnel: w172 -> [w177 _]
              tunnel: w169 -> [w176 _]
              frame True {
                n67 = invoke class="VI" method="FP.Open"(reference=w177, error in=w178, "State"=w176) -> (error out=w179:errorcluster)  [unwired: 2 in, 4 out]
              }
              frame False {
              }
            }
          }
          frame "Maximize", "Maximized" {
            w181 = T3."Maximized" ("State")
            n68 = property class="VI"(error in=w186) -> (reference out=w184:refnum<vi>, error out=w185:errorcluster, "FP.State"=w183:T3)  [unwired: 1 in]
            n69 = Not Equal?(x=w183, y=w181) -> (x != y?=w182:bool)
            n70 = case shown="True" w182 {
              tunnel: [w191 w192] -> w187
              tunnel: w185 -> [w190 w192]
              tunnel: w184 -> [w189 _]
              tunnel: w181 -> [w188 _]
              frame True {
                n71 = invoke class="VI" method="FP.Open"(reference=w189, error in=w190, "State"=w188) -> (error out=w191:errorcluster)  [unwired: 2 in, 4 out]
              }
              frame False {
              }
            }
          }
        }
        n72 = call <vilib>:"Add State(s) to Queue__jki_lib_state_machine.vi"("State(s) in (\"\")"=w132) -> ("States Out"=w131:string)  [unwired: 14 in]
      }
      frame "---------- Macro ----------" {
        # "Do not put any code in this frame.\n(It is a separator no-op. You can make a copy of this frame to create a new Macro frame)"
        n73 = call <vilib>:"Add State(s) to Queue__jki_lib_state_machine.vi"("State(s) in (\"\")"=w196) -> ("States Out"=w195:string)  [unwired: 14 in]
      }
      frame "Macro: Initialize" {
        # "Initialization Macro\n(This is called once, when the VI starts)"
        n74 = call <vilib>:"Add State(s) to Queue__jki_lib_state_machine.vi"("State(s) in Front (\"\")"="Data: Initialize\nInitialize Core Data\nUI: Initialize\nUI: Front Panel State >> Open", "State(s) in (\"\")"=w201) -> ("States Out"=w200:string)  [unwired: 13 in]
      }
      frame "Macro: Exit" {
        # "Exit Macro\n(This is called once, when the VI exits)"
        n75 = disable-structure shown="Enabled" {
          disable-tunnel: w208 -> [w213 _]
          disable-tunnel: [w212 FALSE ("Close Panel on Exit?")] -> w203
          frame Disabled {
            n76 = Unbundle By Name(w213) -> ("Core.Close Panel on Exit?"=w212:bool)
          }
          frame Enabled {
          }
        }
        n77 = Select(t="UI: Front Panel State >> Close", s=w203, f="") -> (s? t:f=w206:string)
        n78 = call <vilib>:"Add State(s) to Queue__jki_lib_state_machine.vi"("State(s) in (\"\")"=w206, "State(s) at Back (\"\")"="Data: Cleanup\nExit") -> ("States Out"=w204:string)  [unwired: 13 in]
        n79 = call <vilib>:"Add State(s) to Queue__jki_lib_state_machine.vi"("State(s) in Front (\"\")"=w204, "State(s) in (\"\")"=w211) -> ("States Out"=w210:string)  [unwired: 13 in]
      }
      frame "---------- Action ----------" {
        # "Do not put any code in this frame.\n(It is a separator no-op. You can make a copy of this frame to create a new Macro frame)"
        n80 = call <vilib>:"Add State(s) to Queue__jki_lib_state_machine.vi"("State(s) in (\"\")"=w218) -> ("States Out"=w217:string)  [unwired: 14 in]
      }
    }
  }
